vi "CC Set Device By Name.vi"(8 "error in (no error)":errorcluster, 10 "Device Name":string, 11 "Device Type":string) -> (0 "error out":errorcluster, 2 "Hardware Config out":T1)   [LabVIEW 2024]
uses:
  typedefs/CC cluster Hardware Config.ctl
  typedefs/CC cluster Device Index.ctl
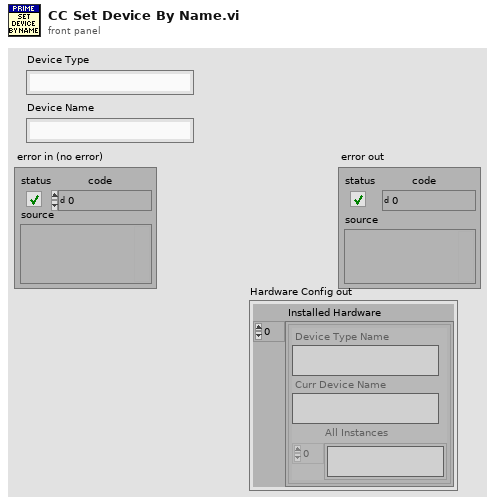
[diagram p1: front panel]
types:
  T1 = typedef "CC cluster Hardware Config.ctl" = cluster{"Installed Hardware":T2[]}
  T2 = typedef "CC cluster Device Index.ctl" = cluster{"Device Type Name":string, "Curr Device Name":string, "All Instances":string[]}
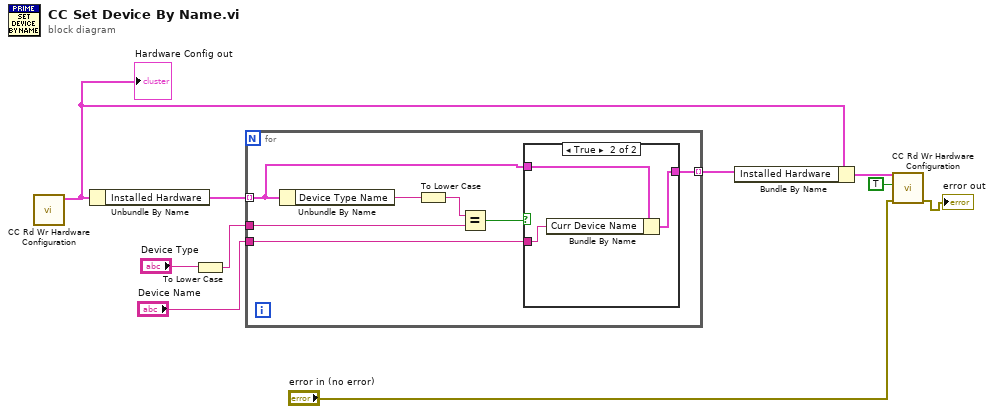
[diagram p0: block diagram]
diagram:
  n1 = call "CC Rd Wr Hardware Configuration.vi"() -> ("Hardware Config out"=w6:T1)  [unwired: 9 in, 2 out]
  "Hardware Config out" <- w6
  n2 = Unbundle By Name(w6) -> ("Installed Hardware"=w10:T2[])
  n3 = To Lower Case(string="Device Type") -> (all lower case string=w8:string)
  n4 = for {
    tunnel: w10 -> [w13] mode=indexing
    tunnel: w8 -> [w15]
    tunnel: [w12] -> w5 mode=indexing
    tunnel: "Device Name" -> [w11]
    n5 = Unbundle By Name(w13) -> ("Device Type Name"=w17:string)
    n6 = To Lower Case(string=w17) -> (all lower case string=w16:string)
    n7 = Equal?(x=w16, y=w15) -> (x = y?=w14:bool)
    n8 = case shown="True" w14 {
      tunnel: w13 -> [w18 w21]
      tunnel: [w18 w19] -> w12
      tunnel: w11 -> [_ w20]
      frame False {
      }
      frame True {
        n9 = Bundle By Name(cluster=w21, "Curr Device Name"=w20) -> (w19:T2)
      }
    }
  }
  n10 = Bundle By Name(cluster=w6, "Installed Hardware"=w5) -> (w4:T1)
  n11 = call "CC Rd Wr Hardware Configuration.vi"("error in (no error)"="error in (no error)", "Write? (F:Read)"=TRUE, "Hardware Config"=w4) -> ("error out"=→"error out":errorcluster)  [unwired: 6 in, 2 out]
